vi "Create User Events.vi"(8 "error in":errorcluster) -> (0 "error out":errorcluster, 3 "User Events":T1)   [LabVIEW 2020, in "User Events.lvlib"]
doc: "Create a boolean user event that will be used to stop the event loop from the message handling loop."
uses:
  User Events.lvlib
  User Events Refs--cluster.ctl
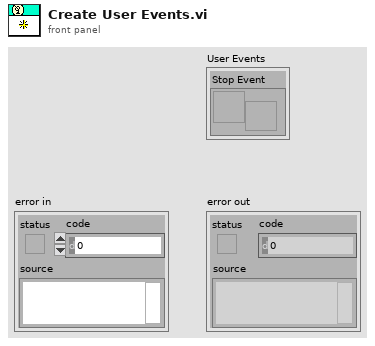
[diagram p1: front panel]
types:
  T1 = typedef "User Events.lvlib/User Events Refs--cluster.ctl" = cluster{"Stop Event":refnum<user-event>}
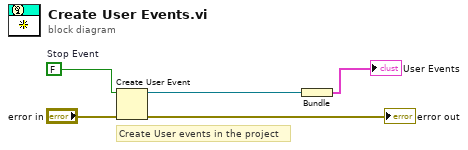
[diagram p0: block diagram]
diagram:
  w2 = FALSE  # Stop Event
  # "Create User events in the project"
  n1 = Create User Event(user event datatype=w2, error in="error in") -> (user event=w1:refnum<user-event>, error out=→"error out":errorcluster)
  n2 = Bundle("Stop Event"=w1) -> (→"User Events":cluster{"Stop Event":refnum<user-event>})  [unwired: 1 in]
